vi "Configure Range Table (Spurious Emissions - Frequency, VBW and RBW).vi"(0 "VISA resource name":refnum<visa-resource-name>, 1 "Auto Resolution Bandwidth List":bool[](array[boolean])=[FALSE, FALSE], 2 "Auto Video Bandwidth List":bool[](array[boolean])=[TRUE, TRUE], 5 "Enable Range List":bool[](array[boolean])=[TRUE, TRUE], 7 "Start Frequency List":dbl[](array[numeric])=[1900000000.0, 1900000000.0], 9 "Stop Frequency List":dbl[](array[numeric])=[2000000000.0, 2000000000.0], 11 "error in (no error)":errorcluster, 12 "Manual Resolution Bandwidth List":dbl[](array[numeric])=[510000.0, 510000.0], 13 "Manual Video Bandwidth List":dbl[](array[numeric])=[51000.0, 51000.0]) -> (4 "VISA resource name out":refnum<visa-resource-name>, 15 "error out":errorcluster)   [LabVIEW 2018, in "Agilent MXA Series.lvlib"]
doc: "Configures the Frequency, VBW and RBW settings under Range Table for Spurious Emissions measurement type."
uses:
  Agilent MXA Series.lvlib
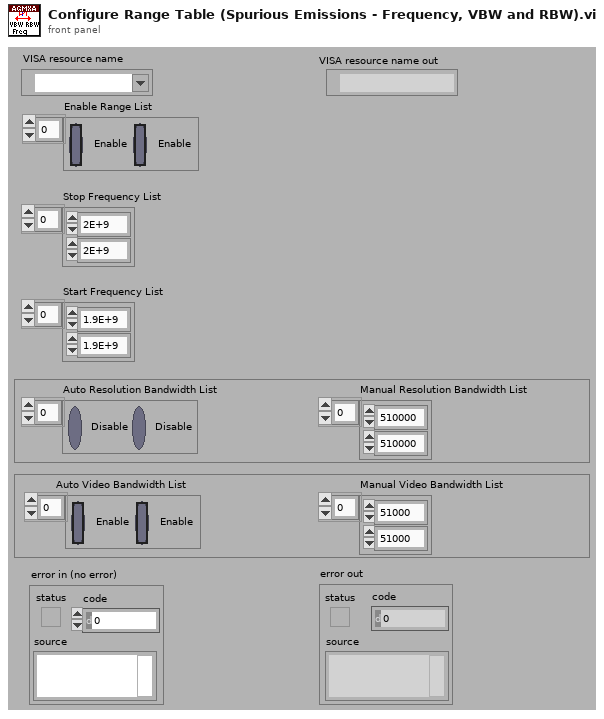
[diagram p1: front panel]
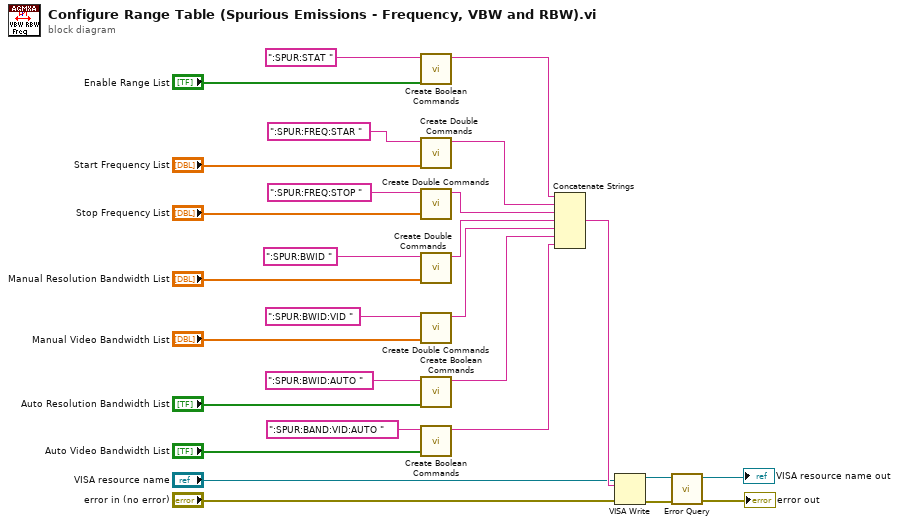
[diagram p0: block diagram]
diagram:
  n1 = call "Create Boolean Commands.vi"("Boolean States"="Enable Range List", "Command"=":SPUR:STAT ") -> ("Result String"=w14:string)  [unwired: 9 in]
  n2 = call "Create Double Commands.vi"("Double Values"="Start Frequency List", "Commands"=":SPUR:FREQ:STAR ") -> ("Result"=w13:string)  [unwired: 9 in]
  n3 = call "Create Double Commands.vi"("Double Values"="Stop Frequency List", "Commands"=":SPUR:FREQ:STOP ") -> ("Result"=w12:string)  [unwired: 9 in]
  n4 = call "Create Double Commands.vi"("Double Values"="Manual Resolution Bandwidth List", "Commands"=":SPUR:BWID ") -> ("Result"=w11:string)  [unwired: 9 in]
  n5 = call "Create Double Commands.vi"("Double Values"="Manual Video Bandwidth List", "Commands"=":SPUR:BWID:VID ") -> ("Result"=w10:string)  [unwired: 9 in]
  n6 = call "Create Boolean Commands.vi"("Boolean States"="Auto Resolution Bandwidth List", "Command"=":SPUR:BWID:AUTO ") -> ("Result String"=w9:string)  [unwired: 9 in]
  n7 = call "Create Boolean Commands.vi"("Boolean States"="Auto Video Bandwidth List", "Command"=":SPUR:BAND:VID:AUTO ") -> ("Result String"=w8:string)  [unwired: 9 in]
  n8 = Concatenate Strings(w14, w13, w12, w11, w10, w9, w8) -> (w7:string)
  n9 = VISA Write(VISA resource name="VISA resource name", write buffer=w7, error in (no error)="error in (no error)") -> (VISA resource name out=w3:refnum<visa-resource-name>, error out=w4:errorcluster)  [unwired: 1 out]
  n10 = call "Error Query.vi"("error in (no error)"=w4, "VISA resource name"=w3) -> ("error out"=→"error out":errorcluster, "VISA resource name out"=→"VISA resource name out":refnum<visa-resource-name>)  [unwired: 6 in, 2 out]
